vi "总磷总氮测量数据储存.vi"   [LabVIEW 2016, in "斯坦道氨氮.lvlib"]
types:
  T1 = enum16{"水样测试", "标样核查", "跨度核查", "零点核查", "加标回收", "空白测试", "平行样"}
  T2 = enum16{"维护数据", "水样测试", "标样核查", "零点核查", "跨度核查", "空白测试", "平行样测试", "加标回收", "空白校准", "标样校准", "初始化（清洗）"}
  T3 = cluster{"时间标识":timestamp, "测量模式":enum16{"维护数据", "水样测试", "标样核查", "零点核查", "跨度核查", "空白测试", "平行样测试", "加标回收", "空白校准", "标样校准", "初始化（清洗）"}, "数据标记表":string, "监测值":sgl, "单位":u16, "数据标识":string, "因子编码":u32, "标样参考值":sgl, "F0":sgl, "F1":sgl, "F2":sgl, "F3":sgl, "F4":sgl, "F5":sgl, "F6":sgl, "F7":sgl, "X":sgl, "温度":sgl, "湿度":sgl, "量程标识":string, "SN":string, "跨度值":sgl}
  T4 = cluster{"运行模式":enum16{"维护模式", "常规模式", "应急模式", "质控模式"}, "质控频次":enum16{"关闭", "每天", "星期一", "星期二", "星期三", "星期四", "星期五", "星期六", "星期日"}, "空白核查时间":u16, "跨度核查时间":u16, "24H周期设置":bool[]}
  T5 = cluster{"系统时间":timestamp, "工作状态":u16, "测量模式":enum16{"待机", "连续模式", "周期模式", "定点模式", "受控模式", "手动模式"}, "告警代码":u16, "故障代码":u16, "日志代码":u16, "软件版本":u16, "F0":sgl, "F1":sgl, "F2":sgl, "F3":sgl, "T":sgl, "H":sgl, "id":u16, "flowid":u16, "量程":u16, "总磷控温温度1":sgl, "营养盐控温温度2":sgl, "ADC":sgl}
  T6 = cluster{"因子编码":u32, "单位":u16, "标样参考值":sgl, "水样数据时间":timestamp, "水样实测值":sgl, "水样数据标识":string, "标样数据时间":timestamp, "标样实测值":sgl, "标样数据标识":string, "空白数据时间":timestamp, "空白实测值":sgl, "空白数据标识":string, "零点核查数据时间":timestamp, "零点核查实测值":sgl, "零点核查数据标识":string, "跨度核查数据时间":timestamp, "跨度核查实测值":sgl, "跨度核查数据标识":string, "加标回收数据时间":timestamp, "加标回收实测值":sgl, "加标回收数据标识":string, "平行样数据时间":timestamp, "平行样实测值":sgl, "平行样数据标识":string, "F0":sgl, "F1":sgl, "F2":sgl, "F3":sgl, "F4":sgl, "F5":sgl, "F6":sgl, "F7":sgl, "温度":sgl, "湿度":sgl, "X值":sgl, "fidrange":u16}[]
  T7 = cluster{"因子编码":u32, "单位":u16, "标样参考值":sgl, "水样数据时间":timestamp, "水样实测值":sgl, "水样数据标识":string, "标样数据时间":timestamp, "标样实测值":sgl, "标样数据标识":string, "空白数据时间":timestamp, "空白实测值":sgl, "空白数据标识":string, "零点核查数据时间":timestamp, "零点核查实测值":sgl, "零点核查数据标识":string, "跨度核查数据时间":timestamp, "跨度核查实测值":sgl, "跨度核查数据标识":string, "加标回收数据时间":timestamp, "加标回收实测值":sgl, "加标回收数据标识":string, "平行样数据时间":timestamp, "平行样实测值":sgl, "平行样数据标识":string, "F0":sgl, "F1":sgl, "F2":sgl, "F3":sgl, "F4":sgl, "F5":sgl, "F6":sgl, "F7":sgl, "温度":sgl, "湿度":sgl, "X值":sgl, "fidrange":u16}
  T8 = cluster{"总磷跨度值":dbl, "总磷零点标准液浓度":dbl, "总磷跨度标准液浓度":dbl, "总磷标准液标准浓度":dbl, "总氮跨度值":dbl, "总氮零点标准液浓度":dbl, "总氮跨度标准液浓度":dbl, "总氮标准液标准浓度":dbl, "COD跨度值":dbl, "COD零点标准液浓度":dbl, "COD跨度标准液浓度":dbl, "COD标准液标准浓度":dbl, "氨氮跨度值":dbl, "氨氮零点标准液浓度":dbl, "氨氮跨度标准液浓度":dbl, "氨氮标准液标准浓度":dbl, "磷酸盐跨度值":dbl, "磷酸盐零点标准液浓度":dbl, "磷酸盐跨度标准液浓度":dbl, "磷酸盐标准液标准浓度":dbl, "硝氮跨度值":dbl, "硝氮零点标准液浓度":dbl, "硝氮跨度标准液浓度":dbl, "硝氮标准液标准浓度":dbl, "亚硝氮跨度值":dbl, "亚硝氮零点标准液浓度":dbl, "亚硝氮跨度标准液浓度":dbl, "亚硝氮标准液标准浓度":dbl, "硫化物跨度值":dbl, "硫化物零点标准液浓度":dbl, "硫化物跨度标准液浓度":dbl, "硫化物标准液标准浓度":dbl, "硅酸盐跨度值":dbl, "硅酸盐零点标准液浓度":dbl, "硅酸盐跨度标准液浓度":dbl, "硅酸盐标准液标准浓度":dbl}
  T9 = typedef "斯坦道氨氮.lvlib/关键参数.ctl" = cluster{"测量量程":sgl, "测量检出限":sgl, "测量精度":sgl, "测量间隔":sgl, "消解温度":sgl, "消解时长":sgl, "三项式系数":sgl, "二次多项式系数":sgl, "曲线斜率":sgl, "曲线截距":sgl, "线性相关系数":sgl, "空白校准时间":timestamp, "标样校准时间":timestamp, "测量信号值":sgl, "稀释倍数":sgl, "量程系数":sgl}
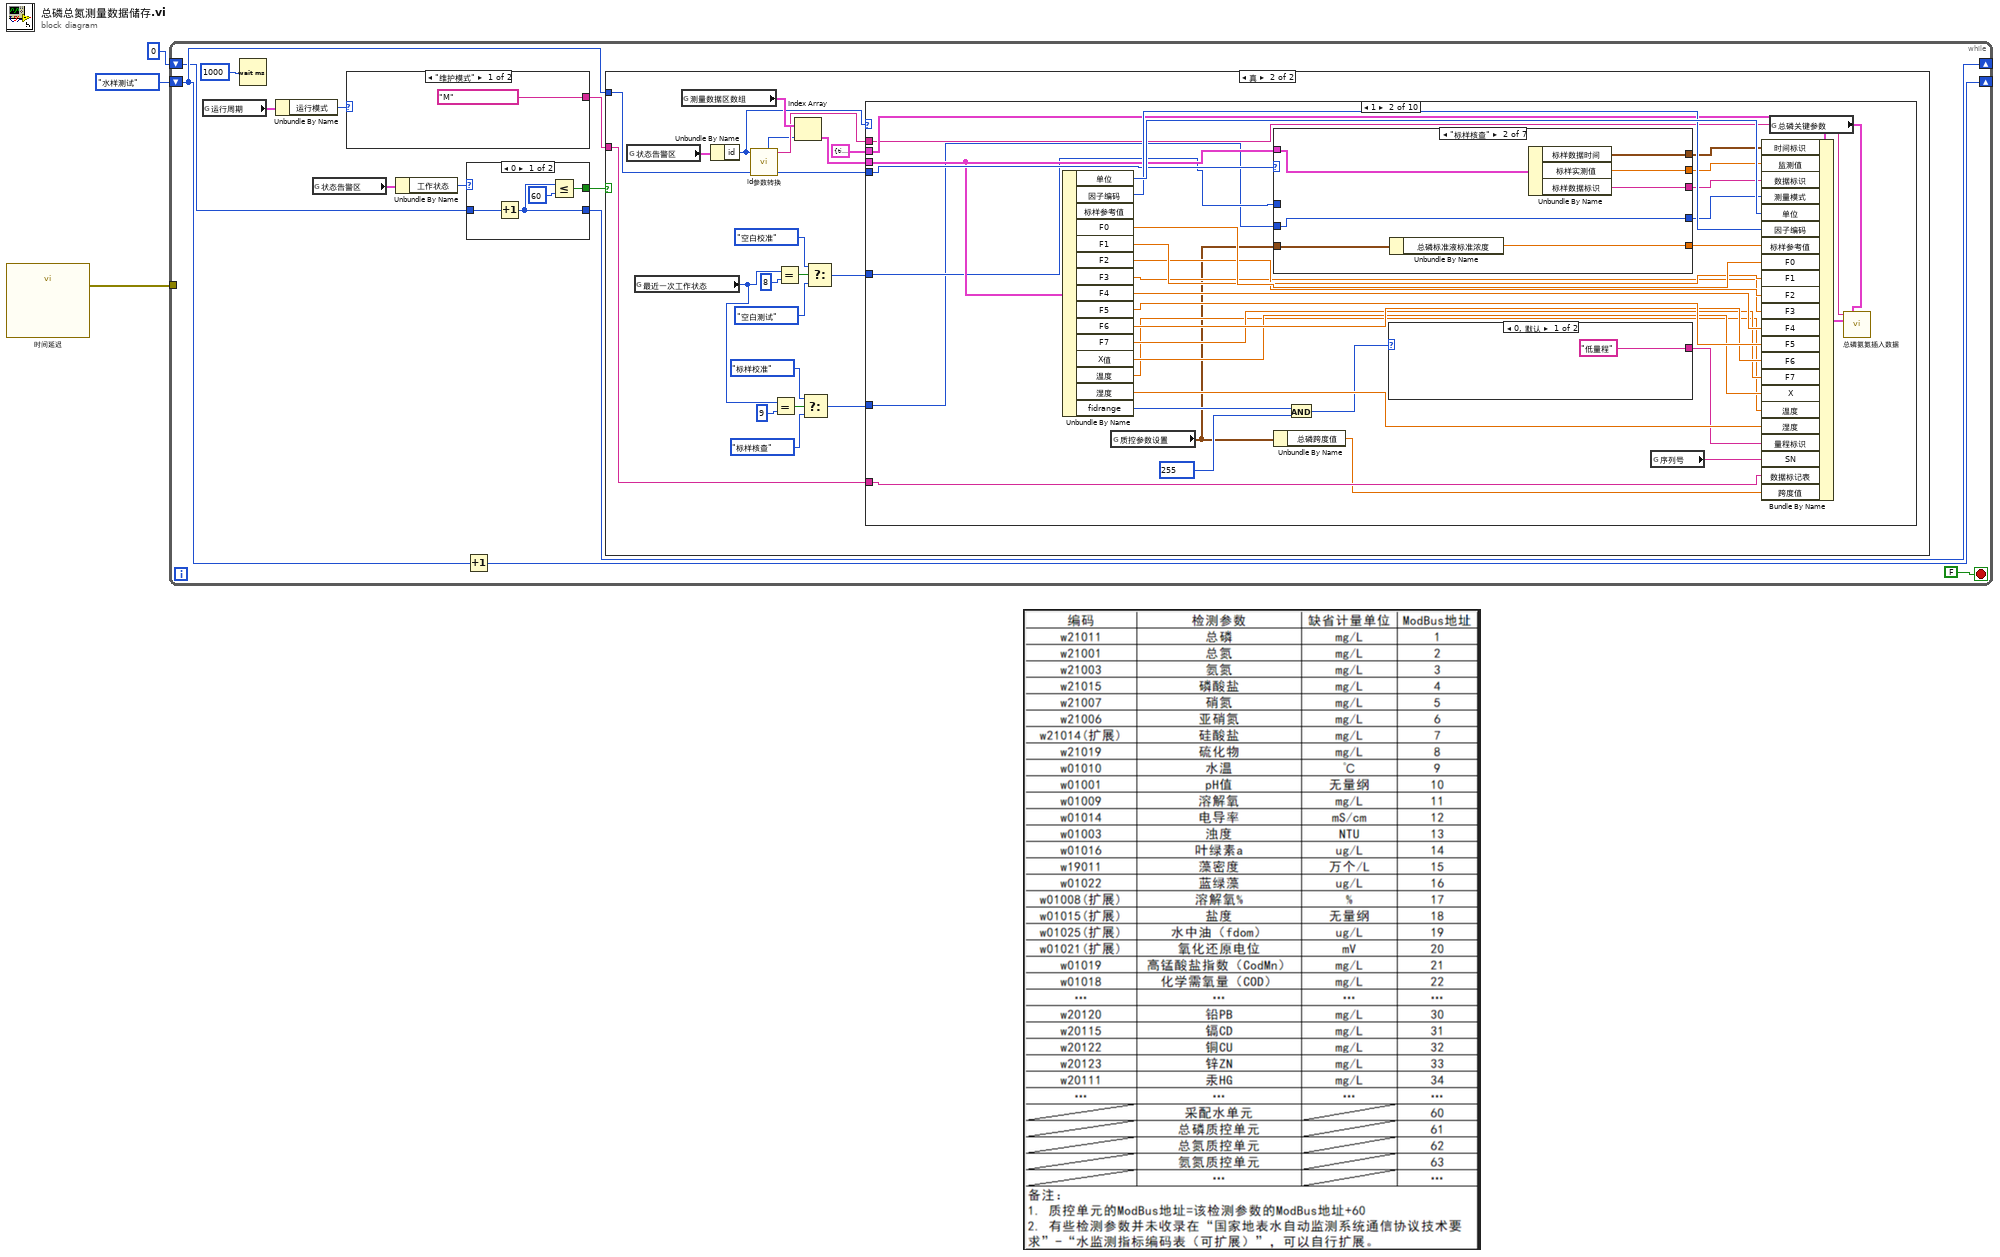
[diagram p0: block diagram]
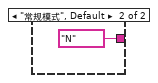
[diagram p3: hidden frame]
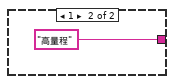
[diagram p6: hidden frame]
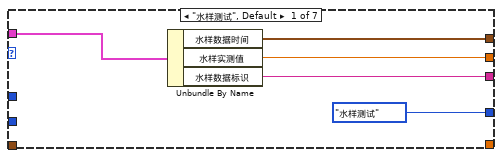
[diagram p7: hidden frame]
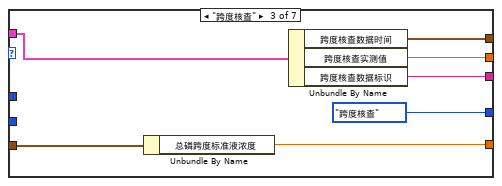
[diagram p8: hidden frame]
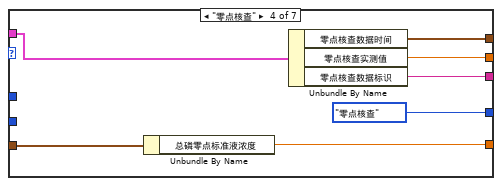
[diagram p9: hidden frame]
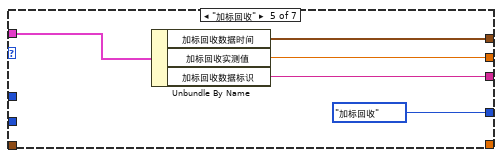
[diagram p10: hidden frame]
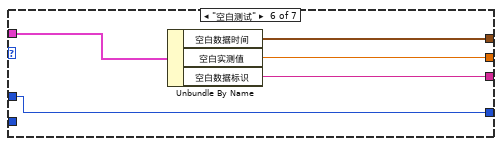
[diagram p11: hidden frame]
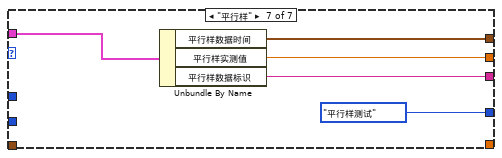
[diagram p12: hidden frame]
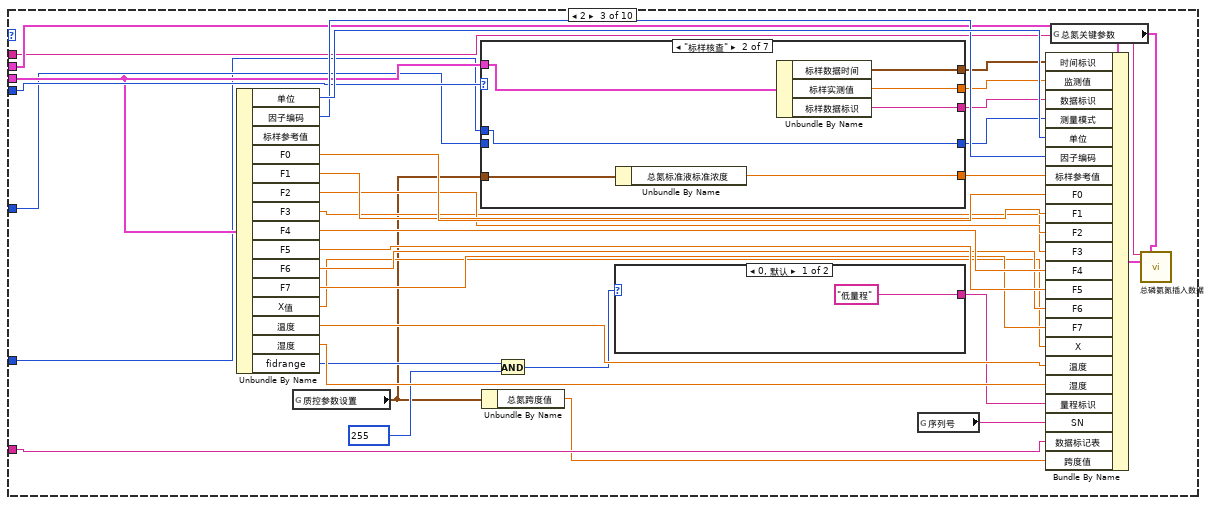
[diagram p13: hidden frame]
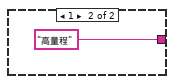
[diagram p14: hidden frame]
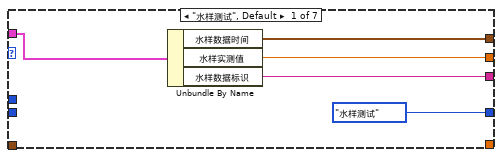
[diagram p15: hidden frame]
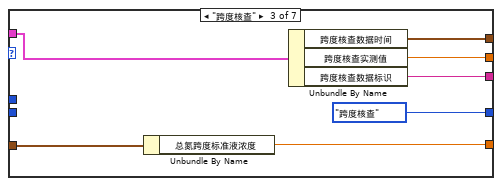
[diagram p16: hidden frame]
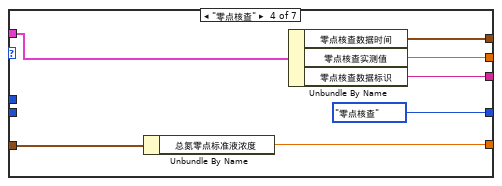
[diagram p17: hidden frame]
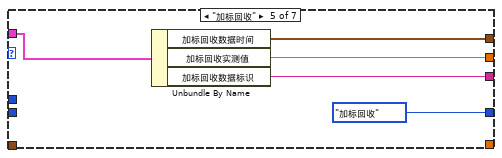
[diagram p18: hidden frame]
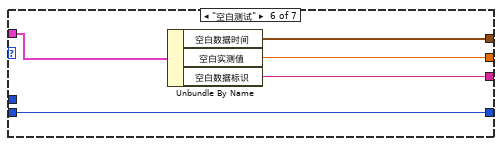
[diagram p19: hidden frame]
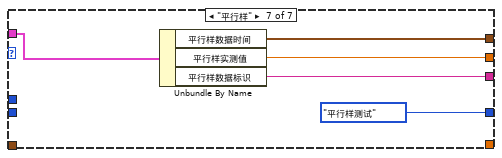
[diagram p20: hidden frame]
diagram:
  n1 = call "时间延迟"() -> ("error out"=w1:errorcluster)  [unwired: 11 in]
  n2 = while {
    shift-right: [w13] -> _
    shift-left: T1."水样测试" ("测量模式") -> [w12]
    shift-right: [w6] -> _
    shift-left: u32 0 ("等待时间（毫秒）") -> [w7]
    tunnel: w1 -> [_]
    stop <- FALSE stop-if-true
    n3 = global read "总磷总氮断电保存全局变量.vi" "运行周期"() -> (w11:T4)
    n4 = Wait (ms)(milliseconds to wait=u32 1000 ("等待时间（毫秒）")) -> ()  [unwired: 1 out]
    n5 = Unbundle By Name(w11) -> ("运行模式"=w10:enum16{"维护模式", "常规模式", "应急模式", "质控模式"})
    n6 = global read "VAR总磷总氮全局变量.vi" "状态告警区"() -> (w9:T5)
    n7 = case shown="\"维护模式\"" w10 {
      tunnel: ["M" ("数据标记表") "N" ("数据标记表")] -> w14
      frame "维护模式" {
      }
      frame "常规模式", Default {
      }
    }
    n8 = Unbundle By Name(w9) -> ("工作状态"=w8:u16)
    n9 = Increment(x=w12) -> (x+1=w13:T1)
    n10 = case shown="0" w8 {
      tunnel: w7 -> [w19 _]
      tunnel: [w18 _] -> w6
      tunnel: [w16 _] -> w5
      frame 0 {
        n11 = Increment(x=w19) -> (x+1=w18:u32)
        n12 = Less Or Equal?(x=w18, y=u32 60) -> (x <= y?=w16:bool)
      }
      frame 1, Default {
      }
    }
    n13 = case shown="真" w5 {
      tunnel: w14 -> [_ w41]
      tunnel: w12 -> [_ w40]
      frame False {
      }
      frame True {
        n14 = global read "VAR总磷总氮全局变量.vi" "状态告警区"() -> (w39:T5)
        n15 = global read "VAR总磷总氮全局变量.vi" "最近一次工作状态"() -> (w24:u16)
        n16 = global read "VAR总磷总氮全局变量.vi" "测量数据区数组"() -> (w37:T6)
        n17 = Unbundle By Name(w39) -> ("id"=w35:u16)
        n18 = call "id参数转换.vi"("id"=w35) -> ("table输出"=w34:string, "数组资源索引"=w33:i32)  [unwired: 9 in]
        n19 = Equal?(x=w24, y=u16 9) -> (x = y?=w26:bool)
        n20 = Equal?(x=w24, y=u16 8) -> (x = y?=w31:bool)
        n21 = Index Array(array=w37, index=w33) -> (element=w36:T7)
        n22 = Select(t=T2."标样校准" ("测量模式"), s=w26, f=T2."标样核查" ("测量模式")) -> (s? t:f=w22:T2)
        n23 = Select(t=T2."空白校准" ("测量模式"), s=w31, f=T2."空白测试" ("测量模式")) -> (s? t:f=w23:T2)
        n24 = case shown="1" w35 {
          tunnel: w41 -> [_ w51 w128 w206 w283 w360 w437 w514 w591 w668]
          tunnel: w40 -> [_ w59 w139 w216 w293 w370 w447 w524 w601 w678]
          tunnel: T3 {"时间标识"=timestamp(0 s since 1904-01-01), "测量模式"=enum."水样测试", "数据标记表"="N", "监测值"=0.0, "单位"=0, "数据标识"="", "因子编码"=0, "标样参考值"=0.0, "F0"=0.0, "F1"=0.0, "F2"=0.0, "F3"=0.0, "F4"=0.0, "F5"=0.0, "F6"=0.0, "F7"=0.0, "X"=0.0, "温度"=0.0, "湿度"=0.0, "量程标识"="", "SN"="", "跨度值"=0.0} ("data") -> [_ w49 w126 w204 w281 w358 w435 w512 w589 w666]
          tunnel: w36 -> [_ w46 w123 w201 w278 w355 w432 w509 w586 w662]
          tunnel: w34 -> [_ w45 w122 w199 w276 w353 w430 w507 w584 w661]
          tunnel: w23 -> [_ w44 w121 w197 w275 w352 w429 w505 w583 w660]
          tunnel: w22 -> [_ w43 w120 w198 w274 w351 w428 w506 w582 w659]
          frame Default {
          }
          frame 1 {
            n25 = Unbundle By Name(w46) -> ("单位"=w75:u16, "因子编码"=w74:u32, "F0"=w73:sgl, "F1"=w72:sgl, "F2"=w71:sgl, "F3"=w70:sgl, "F4"=w69:sgl, "F5"=w68:sgl, "F6"=w67:sgl, "F7"=w66:sgl, "X值"=w65:sgl, "温度"=w64:sgl, "湿度"=w63:sgl, "fidrange"=w57:u16)  [unwired: 1 out]
            n26 = global read "总磷总氮断电保存全局变量.vi" "质控参数设置"() -> (w48:T8)
            n27 = case shown="\"标样核查\"" w59 {
              tunnel: w46 -> [w82 w89 w96 w103 w108 w113 w118]
              tunnel: [w81 w88 w95 w102 w107 w112 w117] -> w60
              tunnel: [w80 w87 w94 w101 w106 w111 w116] -> w61
              tunnel: [w79 w86 w93 w100 w105 w110 w115] -> w62
              tunnel: [T2."水样测试" ("测量模式") w83 T2."跨度核查" ("测量模式") T2."零点核查" ("测量模式") T2."加标回收" ("测量模式") w109 T2."平行样测试" ("测量模式")] -> w50
              tunnel: w48 -> [_ w85 w91 w98 _ _ _]
              tunnel: [_ w84 w90 w97 _ _ _] -> w58
              tunnel: w44 -> [_ _ _ _ _ w109 _]
              tunnel: w43 -> [_ w83 _ _ _ _ _]
              frame "水样测试", Default {
                n28 = Unbundle By Name(w82) -> ("水样数据时间"=w81:timestamp, "水样实测值"=w80:sgl, "水样数据标识"=w79:string)
              }
              frame "标样核查" {
                n29 = Unbundle By Name(w85) -> ("总磷标准液标准浓度"=w84:dbl)
                n30 = Unbundle By Name(w89) -> ("标样数据时间"=w88:timestamp, "标样实测值"=w87:sgl, "标样数据标识"=w86:string)
              }
              frame "跨度核查" {
                n31 = Unbundle By Name(w91) -> ("总磷跨度标准液浓度"=w90:dbl)
                n32 = Unbundle By Name(w96) -> ("跨度核查数据时间"=w95:timestamp, "跨度核查实测值"=w94:sgl, "跨度核查数据标识"=w93:string)
              }
              frame "零点核查" {
                n33 = Unbundle By Name(w98) -> ("总磷零点标准液浓度"=w97:dbl)
                n34 = Unbundle By Name(w103) -> ("零点核查数据时间"=w102:timestamp, "零点核查实测值"=w101:sgl, "零点核查数据标识"=w100:string)
              }
              frame "加标回收" {
                n35 = Unbundle By Name(w108) -> ("加标回收数据时间"=w107:timestamp, "加标回收实测值"=w106:sgl, "加标回收数据标识"=w105:string)
              }
              frame "空白测试" {
                n36 = Unbundle By Name(w113) -> ("空白数据时间"=w112:timestamp, "空白实测值"=w111:sgl, "空白数据标识"=w110:string)
              }
              frame "平行样" {
                n37 = Unbundle By Name(w118) -> ("平行样数据时间"=w117:timestamp, "平行样实测值"=w116:sgl, "平行样数据标识"=w115:string)
              }
            }
            n38 = Unbundle By Name(w48) -> ("总磷跨度值"=w47:dbl)
            n39 = And(x=w57, y=u16 255) -> (x .and. y?=w55:u16)
            n40 = case shown="0, 默认" w55 {
              tunnel: ["低量程" ("格式字符串") "高量程" ("格式字符串")] -> w54
              frame 0, Default {
              }
              frame 1 {
              }
            }
            n41 = global read "VAR总磷总氮全局变量.vi" "序列号"() -> (w52:string)
            n42 = Bundle By Name(cluster=w49, "时间标识"=w60, "监测值"=w61, "数据标识"=w62, "测量模式"=w50, "单位"=w75, "因子编码"=w74, "标样参考值"=w58, "F0"=w73, "F1"=w72, "F2"=w71, "F3"=w70, "F4"=w69, "F5"=w68, "F6"=w67, "F7"=w66, "X"=w65, "温度"=w64, "湿度"=w63, "量程标识"=w54, "SN"=w52, "数据标记表"=w51, "跨度值"=w47) -> (w53:T3)
            n43 = global read "VAR总磷总氮全局变量.vi" "总磷关键参数"() -> (w42:T9)
            n44 = call "总磷氨氮插入数据.vi"("table"=w45, "关键参数"=w42, "data"=w53) -> ()  [unwired: 12 in, 1 out]
          }
          frame 2 {
            n45 = Unbundle By Name(w123) -> ("单位"=w152:u16, "因子编码"=w151:u32, "F0"=w150:sgl, "F1"=w149:sgl, "F2"=w148:sgl, "F3"=w147:sgl, "F4"=w146:sgl, "F5"=w145:sgl, "F6"=w144:sgl, "F7"=w143:sgl, "X值"=w142:sgl, "温度"=w141:sgl, "湿度"=w140:sgl, "fidrange"=w132:u16)  [unwired: 1 out]
            n46 = global read "总磷总氮断电保存全局变量.vi" "质控参数设置"() -> (w125:T8)
            n47 = case shown="\"标样核查\"" w139 {
              tunnel: w123 -> [w159 w166 w173 w180 w185 w190 w195]
              tunnel: [w158 w165 w172 w179 w184 w189 w194] -> w138
              tunnel: [w157 w164 w171 w178 w183 w188 w193] -> w137
              tunnel: [w156 w163 w170 w177 w182 w187 w192] -> w136
              tunnel: [T2."水样测试" ("测量模式") w160 T2."跨度核查" ("测量模式") T2."零点核查" ("测量模式") T2."加标回收" ("测量模式") w186 T2."平行样测试" ("测量模式")] -> w127
              tunnel: w125 -> [_ w162 w168 w175 _ _ _]
              tunnel: [_ w161 w167 w174 _ _ _] -> w135
              tunnel: w121 -> [_ _ _ _ _ w186 _]
              tunnel: w120 -> [_ w160 _ _ _ _ _]
              frame "水样测试", Default {
                n48 = Unbundle By Name(w159) -> ("水样数据时间"=w158:timestamp, "水样实测值"=w157:sgl, "水样数据标识"=w156:string)
              }
              frame "标样核查" {
                n49 = Unbundle By Name(w162) -> ("总氮标准液标准浓度"=w161:dbl)
                n50 = Unbundle By Name(w166) -> ("标样数据时间"=w165:timestamp, "标样实测值"=w164:sgl, "标样数据标识"=w163:string)
              }
              frame "跨度核查" {
                n51 = Unbundle By Name(w168) -> ("总氮跨度标准液浓度"=w167:dbl)
                n52 = Unbundle By Name(w173) -> ("跨度核查数据时间"=w172:timestamp, "跨度核查实测值"=w171:sgl, "跨度核查数据标识"=w170:string)
              }
              frame "零点核查" {
                n53 = Unbundle By Name(w175) -> ("总氮零点标准液浓度"=w174:dbl)
                n54 = Unbundle By Name(w180) -> ("零点核查数据时间"=w179:timestamp, "零点核查实测值"=w178:sgl, "零点核查数据标识"=w177:string)
              }
              frame "加标回收" {
                n55 = Unbundle By Name(w185) -> ("加标回收数据时间"=w184:timestamp, "加标回收实测值"=w183:sgl, "加标回收数据标识"=w182:string)
              }
              frame "空白测试" {
                n56 = Unbundle By Name(w190) -> ("空白数据时间"=w189:timestamp, "空白实测值"=w188:sgl, "空白数据标识"=w187:string)
              }
              frame "平行样" {
                n57 = Unbundle By Name(w195) -> ("平行样数据时间"=w194:timestamp, "平行样实测值"=w193:sgl, "平行样数据标识"=w192:string)
              }
            }
            n58 = Unbundle By Name(w125) -> ("总氮跨度值"=w124:dbl)
            n59 = And(x=w132, y=u16 255) -> (x .and. y?=w133:u16)
            n60 = case shown="0, 默认" w133 {
              tunnel: ["低量程" ("格式字符串") "高量程" ("格式字符串")] -> w131
              frame 0, Default {
              }
              frame 1 {
              }
            }
            n61 = global read "VAR总磷总氮全局变量.vi" "序列号"() -> (w129:string)
            n62 = Bundle By Name(cluster=w126, "时间标识"=w138, "监测值"=w137, "数据标识"=w136, "测量模式"=w127, "单位"=w152, "因子编码"=w151, "标样参考值"=w135, "F0"=w150, "F1"=w149, "F2"=w148, "F3"=w147, "F4"=w146, "F5"=w145, "F6"=w144, "F7"=w143, "X"=w142, "温度"=w141, "湿度"=w140, "量程标识"=w131, "SN"=w129, "数据标记表"=w128, "跨度值"=w124) -> (w130:T3)
            n63 = global read "VAR总磷总氮全局变量.vi" "总氮关键参数"() -> (w119:T9)
            n64 = call "总磷氨氮插入数据.vi"("table"=w122, "关键参数"=w119, "data"=w130) -> ()  [unwired: 12 in, 1 out]
          }
          frame 3 {
            n65 = Unbundle By Name(w201) -> ("单位"=w229:u16, "因子编码"=w228:u32, "F0"=w227:sgl, "F1"=w226:sgl, "F2"=w225:sgl, "F3"=w224:sgl, "F4"=w223:sgl, "F5"=w222:sgl, "F6"=w221:sgl, "F7"=w220:sgl, "X值"=w219:sgl, "温度"=w218:sgl, "湿度"=w217:sgl, "fidrange"=w209:u16)  [unwired: 1 out]
            n66 = global read "总磷总氮断电保存全局变量.vi" "质控参数设置"() -> (w203:T8)
            n67 = case shown="\"空白测试\"" w216 {
              tunnel: w201 -> [w236 w243 w250 w257 w262 w267 w272]
              tunnel: [w235 w242 w249 w256 w261 w266 w271] -> w215
              tunnel: [w234 w241 w248 w255 w260 w265 w270] -> w214
              tunnel: [w233 w240 w247 w254 w259 w264 w269] -> w213
              tunnel: [T2."水样测试" ("测量模式") w237 T2."跨度核查" ("测量模式") T2."零点核查" ("测量模式") T2."加标回收" ("测量模式") w263 T2."平行样测试" ("测量模式")] -> w205
              tunnel: w203 -> [_ w239 w245 w252 _ _ _]
              tunnel: [_ w238 w244 w251 _ _ _] -> w212
              tunnel: w198 -> [_ w237 _ _ _ _ _]
              tunnel: w197 -> [_ _ _ _ _ w263 _]
              frame "水样测试", Default {
                n68 = Unbundle By Name(w236) -> ("水样数据时间"=w235:timestamp, "水样实测值"=w234:sgl, "水样数据标识"=w233:string)
              }
              frame "标样核查" {
                n69 = Unbundle By Name(w239) -> ("氨氮标准液标准浓度"=w238:dbl)
                n70 = Unbundle By Name(w243) -> ("标样数据时间"=w242:timestamp, "标样实测值"=w241:sgl, "标样数据标识"=w240:string)
              }
              frame "跨度核查" {
                n71 = Unbundle By Name(w245) -> ("氨氮跨度标准液浓度"=w244:dbl)
                n72 = Unbundle By Name(w250) -> ("跨度核查数据时间"=w249:timestamp, "跨度核查实测值"=w248:sgl, "跨度核查数据标识"=w247:string)
              }
              frame "零点核查" {
                n73 = Unbundle By Name(w252) -> ("氨氮零点标准液浓度"=w251:dbl)
                n74 = Unbundle By Name(w257) -> ("零点核查数据时间"=w256:timestamp, "零点核查实测值"=w255:sgl, "零点核查数据标识"=w254:string)
              }
              frame "加标回收" {
                n75 = Unbundle By Name(w262) -> ("加标回收数据时间"=w261:timestamp, "加标回收实测值"=w260:sgl, "加标回收数据标识"=w259:string)
              }
              frame "空白测试" {
                n76 = Unbundle By Name(w267) -> ("空白数据时间"=w266:timestamp, "空白实测值"=w265:sgl, "空白数据标识"=w264:string)
              }
              frame "平行样" {
                n77 = Unbundle By Name(w272) -> ("平行样数据时间"=w271:timestamp, "平行样实测值"=w270:sgl, "平行样数据标识"=w269:string)
              }
            }
            n78 = Unbundle By Name(w203) -> ("氨氮跨度值"=w202:dbl)
            n79 = And(x=w209, y=u16 255) -> (x .and. y?=w210:u16)
            n80 = case shown="0, 默认" w210 {
              tunnel: ["低量程" ("格式字符串") "高量程" ("格式字符串")] -> w208
              frame 0, Default {
              }
              frame 1 {
              }
            }
            n81 = global read "VAR总磷总氮全局变量.vi" "序列号"() -> (w207:string)
            n82 = Bundle By Name(cluster=w204, "时间标识"=w215, "监测值"=w214, "数据标识"=w213, "测量模式"=w205, "单位"=w229, "因子编码"=w228, "标样参考值"=w212, "F0"=w227, "F1"=w226, "F2"=w225, "F3"=w224, "F4"=w223, "F5"=w222, "F6"=w221, "F7"=w220, "X"=w219, "温度"=w218, "湿度"=w217, "量程标识"=w208, "SN"=w207, "数据标记表"=w206, "跨度值"=w202) -> (w200:T3)
            n83 = global read "VAR总磷总氮全局变量.vi" "氨氮关键参数"() -> (w196:T9)
            n84 = call "总磷氨氮插入数据.vi"("table"=w199, "关键参数"=w196, "data"=w200) -> ()  [unwired: 12 in, 1 out]
          }
          frame 4 {
            n85 = Unbundle By Name(w278) -> ("单位"=w306:u16, "因子编码"=w305:u32, "F0"=w304:sgl, "F1"=w303:sgl, "F2"=w302:sgl, "F3"=w301:sgl, "F4"=w300:sgl, "F5"=w299:sgl, "F6"=w298:sgl, "F7"=w297:sgl, "X值"=w296:sgl, "温度"=w295:sgl, "湿度"=w294:sgl, "fidrange"=w286:u16)  [unwired: 1 out]
            n86 = global read "总磷总氮断电保存全局变量.vi" "质控参数设置"() -> (w280:T8)
            n87 = Unbundle By Name(w280) -> ("磷酸盐跨度值"=w279:dbl)
            n88 = case shown="\"标样核查\"" w293 {
              tunnel: w278 -> [w313 w320 w327 w334 w339 w344 w349]
              tunnel: [w312 w319 w326 w333 w338 w343 w348] -> w292
              tunnel: [w311 w318 w325 w332 w337 w342 w347] -> w291
              tunnel: [w310 w317 w324 w331 w336 w341 w346] -> w290
              tunnel: [T2."水样测试" ("测量模式") w314 T2."跨度核查" ("测量模式") T2."零点核查" ("测量模式") T2."加标回收" ("测量模式") w340 T2."平行样测试" ("测量模式")] -> w282
              tunnel: w280 -> [_ w316 w322 w329 _ _ _]
              tunnel: [_ w315 w321 w328 _ _ _] -> w289
              tunnel: w275 -> [_ _ _ _ _ w340 _]
              tunnel: w274 -> [_ w314 _ _ _ _ _]
              frame "水样测试", Default {
                n89 = Unbundle By Name(w313) -> ("水样数据时间"=w312:timestamp, "水样实测值"=w311:sgl, "水样数据标识"=w310:string)
              }
              frame "标样核查" {
                n90 = Unbundle By Name(w316) -> ("磷酸盐标准液标准浓度"=w315:dbl)
                n91 = Unbundle By Name(w320) -> ("标样数据时间"=w319:timestamp, "标样实测值"=w318:sgl, "标样数据标识"=w317:string)
              }
              frame "跨度核查" {
                n92 = Unbundle By Name(w322) -> ("磷酸盐跨度标准液浓度"=w321:dbl)
                n93 = Unbundle By Name(w327) -> ("跨度核查数据时间"=w326:timestamp, "跨度核查实测值"=w325:sgl, "跨度核查数据标识"=w324:string)
              }
              frame "零点核查" {
                n94 = Unbundle By Name(w329) -> ("磷酸盐零点标准液浓度"=w328:dbl)
                n95 = Unbundle By Name(w334) -> ("零点核查数据时间"=w333:timestamp, "零点核查实测值"=w332:sgl, "零点核查数据标识"=w331:string)
              }
              frame "加标回收" {
                n96 = Unbundle By Name(w339) -> ("加标回收数据时间"=w338:timestamp, "加标回收实测值"=w337:sgl, "加标回收数据标识"=w336:string)
              }
              frame "空白测试" {
                n97 = Unbundle By Name(w344) -> ("空白数据时间"=w343:timestamp, "空白实测值"=w342:sgl, "空白数据标识"=w341:string)
              }
              frame "平行样" {
                n98 = Unbundle By Name(w349) -> ("平行样数据时间"=w348:timestamp, "平行样实测值"=w347:sgl, "平行样数据标识"=w346:string)
              }
            }
            n99 = And(x=w286, y=u16 255) -> (x .and. y?=w287:u16)
            n100 = case shown="0, 默认" w287 {
              tunnel: ["低量程" ("格式字符串") "高量程" ("格式字符串")] -> w285
              frame 0, Default {
              }
              frame 1 {
              }
            }
            n101 = global read "VAR总磷总氮全局变量.vi" "序列号"() -> (w284:string)
            n102 = Bundle By Name(cluster=w281, "时间标识"=w292, "监测值"=w291, "数据标识"=w290, "测量模式"=w282, "单位"=w306, "因子编码"=w305, "标样参考值"=w289, "F0"=w304, "F1"=w303, "F2"=w302, "F3"=w301, "F4"=w300, "F5"=w299, "F6"=w298, "F7"=w297, "X"=w296, "温度"=w295, "湿度"=w294, "量程标识"=w285, "SN"=w284, "数据标记表"=w283, "跨度值"=w279) -> (w277:T3)
            n103 = global read "VAR总磷总氮全局变量.vi" "磷酸盐关键参数"() -> (w273:T9)
            n104 = call "总磷氨氮插入数据.vi"("table"=w276, "关键参数"=w273, "data"=w277) -> ()  [unwired: 12 in, 1 out]
          }
          frame 5 {
            n105 = Unbundle By Name(w355) -> ("单位"=w383:u16, "因子编码"=w382:u32, "F0"=w381:sgl, "F1"=w380:sgl, "F2"=w379:sgl, "F3"=w378:sgl, "F4"=w377:sgl, "F5"=w376:sgl, "F6"=w375:sgl, "F7"=w374:sgl, "X值"=w373:sgl, "温度"=w372:sgl, "湿度"=w371:sgl, "fidrange"=w363:u16)  [unwired: 1 out]
            n106 = global read "总磷总氮断电保存全局变量.vi" "质控参数设置"() -> (w357:T8)
            n107 = case shown="\"标样核查\"" w370 {
              tunnel: w355 -> [w390 w397 w404 w411 w416 w421 w426]
              tunnel: [w389 w396 w403 w410 w415 w420 w425] -> w369
              tunnel: [w388 w395 w402 w409 w414 w419 w424] -> w368
              tunnel: [w387 w394 w401 w408 w413 w418 w423] -> w367
              tunnel: [T2."水样测试" ("测量模式") w391 T2."跨度核查" ("测量模式") T2."零点核查" ("测量模式") T2."加标回收" ("测量模式") w417 T2."平行样测试" ("测量模式")] -> w359
              tunnel: w357 -> [_ w393 w399 w406 _ _ _]
              tunnel: [_ w392 w398 w405 _ _ _] -> w366
              tunnel: w352 -> [_ _ _ _ _ w417 _]
              tunnel: w351 -> [_ w391 _ _ _ _ _]
              frame "水样测试", Default {
                n108 = Unbundle By Name(w390) -> ("水样数据时间"=w389:timestamp, "水样实测值"=w388:sgl, "水样数据标识"=w387:string)
              }
              frame "标样核查" {
                n109 = Unbundle By Name(w393) -> ("硝氮标准液标准浓度"=w392:dbl)
                n110 = Unbundle By Name(w397) -> ("标样数据时间"=w396:timestamp, "标样实测值"=w395:sgl, "标样数据标识"=w394:string)
              }
              frame "跨度核查" {
                n111 = Unbundle By Name(w399) -> ("硝氮跨度标准液浓度"=w398:dbl)
                n112 = Unbundle By Name(w404) -> ("跨度核查数据时间"=w403:timestamp, "跨度核查实测值"=w402:sgl, "跨度核查数据标识"=w401:string)
              }
              frame "零点核查" {
                n113 = Unbundle By Name(w406) -> ("硝氮零点标准液浓度"=w405:dbl)
                n114 = Unbundle By Name(w411) -> ("零点核查数据时间"=w410:timestamp, "零点核查实测值"=w409:sgl, "零点核查数据标识"=w408:string)
              }
              frame "加标回收" {
                n115 = Unbundle By Name(w416) -> ("加标回收数据时间"=w415:timestamp, "加标回收实测值"=w414:sgl, "加标回收数据标识"=w413:string)
              }
              frame "空白测试" {
                n116 = Unbundle By Name(w421) -> ("空白数据时间"=w420:timestamp, "空白实测值"=w419:sgl, "空白数据标识"=w418:string)
              }
              frame "平行样" {
                n117 = Unbundle By Name(w426) -> ("平行样数据时间"=w425:timestamp, "平行样实测值"=w424:sgl, "平行样数据标识"=w423:string)
              }
            }
            n118 = Unbundle By Name(w357) -> ("硝氮跨度值"=w356:dbl)
            n119 = And(x=w363, y=u16 255) -> (x .and. y?=w364:u16)
            n120 = case shown="0, 默认" w364 {
              tunnel: ["低量程" ("格式字符串") "高量程" ("格式字符串")] -> w362
              frame 0, Default {
              }
              frame 1 {
              }
            }
            n121 = global read "VAR总磷总氮全局变量.vi" "序列号"() -> (w361:string)
            n122 = Bundle By Name(cluster=w358, "时间标识"=w369, "监测值"=w368, "数据标识"=w367, "测量模式"=w359, "单位"=w383, "因子编码"=w382, "标样参考值"=w366, "F0"=w381, "F1"=w380, "F2"=w379, "F3"=w378, "F4"=w377, "F5"=w376, "F6"=w375, "F7"=w374, "X"=w373, "温度"=w372, "湿度"=w371, "量程标识"=w362, "SN"=w361, "数据标记表"=w360, "跨度值"=w356) -> (w354:T3)
            n123 = global read "VAR总磷总氮全局变量.vi" "硝氮关键参数"() -> (w350:T9)
            n124 = call "总磷氨氮插入数据.vi"("table"=w353, "关键参数"=w350, "data"=w354) -> ()  [unwired: 12 in, 1 out]
          }
          frame 6 {
            n125 = Unbundle By Name(w432) -> ("单位"=w460:u16, "因子编码"=w459:u32, "F0"=w458:sgl, "F1"=w457:sgl, "F2"=w456:sgl, "F3"=w455:sgl, "F4"=w454:sgl, "F5"=w453:sgl, "F6"=w452:sgl, "F7"=w451:sgl, "X值"=w450:sgl, "温度"=w449:sgl, "湿度"=w448:sgl, "fidrange"=w440:u16)  [unwired: 1 out]
            n126 = global read "总磷总氮断电保存全局变量.vi" "质控参数设置"() -> (w434:T8)
            n127 = Unbundle By Name(w434) -> ("亚硝氮跨度值"=w433:dbl)
            n128 = case shown="\"标样核查\"" w447 {
              tunnel: w432 -> [w467 w474 w481 w488 w493 w498 w503]
              tunnel: [w466 w473 w480 w487 w492 w497 w502] -> w446
              tunnel: [w465 w472 w479 w486 w491 w496 w501] -> w445
              tunnel: [w464 w471 w478 w485 w490 w495 w500] -> w444
              tunnel: [T2."水样测试" ("测量模式") w468 T2."跨度核查" ("测量模式") T2."零点核查" ("测量模式") T2."加标回收" ("测量模式") w494 T2."平行样测试" ("测量模式")] -> w436
              tunnel: w434 -> [_ w470 w476 w483 _ _ _]
              tunnel: [_ w469 w475 w482 _ _ _] -> w443
              tunnel: w429 -> [_ _ _ _ _ w494 _]
              tunnel: w428 -> [_ w468 _ _ _ _ _]
              frame "水样测试", Default {
                n129 = Unbundle By Name(w467) -> ("水样数据时间"=w466:timestamp, "水样实测值"=w465:sgl, "水样数据标识"=w464:string)
              }
              frame "标样核查" {
                n130 = Unbundle By Name(w470) -> ("亚硝氮标准液标准浓度"=w469:dbl)
                n131 = Unbundle By Name(w474) -> ("标样数据时间"=w473:timestamp, "标样实测值"=w472:sgl, "标样数据标识"=w471:string)
              }
              frame "跨度核查" {
                n132 = Unbundle By Name(w476) -> ("亚硝氮跨度标准液浓度"=w475:dbl)
                n133 = Unbundle By Name(w481) -> ("跨度核查数据时间"=w480:timestamp, "跨度核查实测值"=w479:sgl, "跨度核查数据标识"=w478:string)
              }
              frame "零点核查" {
                n134 = Unbundle By Name(w483) -> ("亚硝氮零点标准液浓度"=w482:dbl)
                n135 = Unbundle By Name(w488) -> ("零点核查数据时间"=w487:timestamp, "零点核查实测值"=w486:sgl, "零点核查数据标识"=w485:string)
              }
              frame "加标回收" {
                n136 = Unbundle By Name(w493) -> ("加标回收数据时间"=w492:timestamp, "加标回收实测值"=w491:sgl, "加标回收数据标识"=w490:string)
              }
              frame "空白测试" {
                n137 = Unbundle By Name(w498) -> ("空白数据时间"=w497:timestamp, "空白实测值"=w496:sgl, "空白数据标识"=w495:string)
              }
              frame "平行样" {
                n138 = Unbundle By Name(w503) -> ("平行样数据时间"=w502:timestamp, "平行样实测值"=w501:sgl, "平行样数据标识"=w500:string)
              }
            }
            n139 = And(x=w440, y=u16 255) -> (x .and. y?=w441:u16)
            n140 = case shown="0, 默认" w441 {
              tunnel: ["低量程" ("格式字符串") "高量程" ("格式字符串")] -> w439
              frame 0, Default {
              }
              frame 1 {
              }
            }
            n141 = global read "VAR总磷总氮全局变量.vi" "序列号"() -> (w438:string)
            n142 = Bundle By Name(cluster=w435, "时间标识"=w446, "监测值"=w445, "数据标识"=w444, "测量模式"=w436, "单位"=w460, "因子编码"=w459, "标样参考值"=w443, "F0"=w458, "F1"=w457, "F2"=w456, "F3"=w455, "F4"=w454, "F5"=w453, "F6"=w452, "F7"=w451, "X"=w450, "温度"=w449, "湿度"=w448, "量程标识"=w439, "SN"=w438, "数据标记表"=w437, "跨度值"=w433) -> (w431:T3)
            n143 = global read "VAR总磷总氮全局变量.vi" "亚硝氮关键参数"() -> (w427:T9)
            n144 = call "总磷氨氮插入数据.vi"("table"=w430, "关键参数"=w427, "data"=w431) -> ()  [unwired: 12 in, 1 out]
          }
          frame 7 {
            n145 = Unbundle By Name(w509) -> ("单位"=w537:u16, "因子编码"=w536:u32, "F0"=w535:sgl, "F1"=w534:sgl, "F2"=w533:sgl, "F3"=w532:sgl, "F4"=w531:sgl, "F5"=w530:sgl, "F6"=w529:sgl, "F7"=w528:sgl, "X值"=w527:sgl, "温度"=w526:sgl, "湿度"=w525:sgl, "fidrange"=w517:u16)  [unwired: 1 out]
            n146 = global read "总磷总氮断电保存全局变量.vi" "质控参数设置"() -> (w511:T8)
            n147 = Unbundle By Name(w511) -> ("硅酸盐跨度值"=w510:dbl)
            n148 = case shown="\"空白测试\"" w524 {
              tunnel: w509 -> [w544 w551 w558 w565 w570 w575 w580]
              tunnel: [w543 w550 w557 w564 w569 w574 w579] -> w523
              tunnel: [w542 w549 w556 w563 w568 w573 w578] -> w522
              tunnel: [w541 w548 w555 w562 w567 w572 w577] -> w521
              tunnel: [T2."水样测试" ("测量模式") w545 T2."跨度核查" ("测量模式") T2."零点核查" ("测量模式") T2."加标回收" ("测量模式") w571 T2."平行样测试" ("测量模式")] -> w513
              tunnel: w511 -> [_ w547 w553 w560 _ _ _]
              tunnel: [_ w546 w552 w559 _ _ _] -> w520
              tunnel: w506 -> [_ w545 _ _ _ _ _]
              tunnel: w505 -> [_ _ _ _ _ w571 _]
              frame "水样测试", Default {
                n149 = Unbundle By Name(w544) -> ("水样数据时间"=w543:timestamp, "水样实测值"=w542:sgl, "水样数据标识"=w541:string)
              }
              frame "标样核查" {
                n150 = Unbundle By Name(w547) -> ("硅酸盐标准液标准浓度"=w546:dbl)
                n151 = Unbundle By Name(w551) -> ("标样数据时间"=w550:timestamp, "标样实测值"=w549:sgl, "标样数据标识"=w548:string)
              }
              frame "跨度核查" {
                n152 = Unbundle By Name(w553) -> ("硅酸盐跨度标准液浓度"=w552:dbl)
                n153 = Unbundle By Name(w558) -> ("跨度核查数据时间"=w557:timestamp, "跨度核查实测值"=w556:sgl, "跨度核查数据标识"=w555:string)
              }
              frame "零点核查" {
                n154 = Unbundle By Name(w560) -> ("硅酸盐零点标准液浓度"=w559:dbl)
                n155 = Unbundle By Name(w565) -> ("零点核查数据时间"=w564:timestamp, "零点核查实测值"=w563:sgl, "零点核查数据标识"=w562:string)
              }
              frame "加标回收" {
                n156 = Unbundle By Name(w570) -> ("加标回收数据时间"=w569:timestamp, "加标回收实测值"=w568:sgl, "加标回收数据标识"=w567:string)
              }
              frame "空白测试" {
                n157 = Unbundle By Name(w575) -> ("空白数据时间"=w574:timestamp, "空白实测值"=w573:sgl, "空白数据标识"=w572:string)
              }
              frame "平行样" {
                n158 = Unbundle By Name(w580) -> ("平行样数据时间"=w579:timestamp, "平行样实测值"=w578:sgl, "平行样数据标识"=w577:string)
              }
            }
            n159 = And(x=w517, y=u16 255) -> (x .and. y?=w518:u16)
            n160 = case shown="0, 默认" w518 {
              tunnel: ["低量程" ("格式字符串") "高量程" ("格式字符串")] -> w516
              frame 0, Default {
              }
              frame 1 {
              }
            }
            n161 = global read "VAR总磷总氮全局变量.vi" "序列号"() -> (w515:string)
            n162 = Bundle By Name(cluster=w512, "时间标识"=w523, "监测值"=w522, "数据标识"=w521, "测量模式"=w513, "单位"=w537, "因子编码"=w536, "标样参考值"=w520, "F0"=w535, "F1"=w534, "F2"=w533, "F3"=w532, "F4"=w531, "F5"=w530, "F6"=w529, "F7"=w528, "X"=w527, "温度"=w526, "湿度"=w525, "量程标识"=w516, "SN"=w515, "数据标记表"=w514, "跨度值"=w510) -> (w508:T3)
            n163 = global read "VAR总磷总氮全局变量.vi" "硅酸盐关键参数"() -> (w504:T9)
            n164 = call "总磷氨氮插入数据.vi"("table"=w507, "关键参数"=w504, "data"=w508) -> ()  [unwired: 12 in, 1 out]
          }
          frame 8 {
            n165 = Unbundle By Name(w586) -> ("单位"=w614:u16, "因子编码"=w613:u32, "F0"=w612:sgl, "F1"=w611:sgl, "F2"=w610:sgl, "F3"=w609:sgl, "F4"=w608:sgl, "F5"=w607:sgl, "F6"=w606:sgl, "F7"=w605:sgl, "X值"=w604:sgl, "温度"=w603:sgl, "湿度"=w602:sgl, "fidrange"=w594:u16)  [unwired: 1 out]
            n166 = global read "总磷总氮断电保存全局变量.vi" "质控参数设置"() -> (w588:T8)
            n167 = Unbundle By Name(w588) -> ("硫化物跨度值"=w587:dbl)
            n168 = case shown="\"标样核查\"" w601 {
              tunnel: w586 -> [w621 w628 w635 w642 w647 w652 w657]
              tunnel: [w620 w627 w634 w641 w646 w651 w656] -> w600
              tunnel: [w619 w626 w633 w640 w645 w650 w655] -> w599
              tunnel: [w618 w625 w632 w639 w644 w649 w654] -> w598
              tunnel: [T2."水样测试" ("测量模式") w622 T2."跨度核查" ("测量模式") T2."零点核查" ("测量模式") T2."加标回收" ("测量模式") w648 T2."平行样测试" ("测量模式")] -> w590
              tunnel: w588 -> [_ w624 w630 w637 _ _ _]
              tunnel: [_ w623 w629 w636 _ _ _] -> w597
              tunnel: w583 -> [_ _ _ _ _ w648 _]
              tunnel: w582 -> [_ w622 _ _ _ _ _]
              frame "水样测试", Default {
                n169 = Unbundle By Name(w621) -> ("水样数据时间"=w620:timestamp, "水样实测值"=w619:sgl, "水样数据标识"=w618:string)
              }
              frame "标样核查" {
                n170 = Unbundle By Name(w624) -> ("硫化物标准液标准浓度"=w623:dbl)
                n171 = Unbundle By Name(w628) -> ("标样数据时间"=w627:timestamp, "标样实测值"=w626:sgl, "标样数据标识"=w625:string)
              }
              frame "跨度核查" {
                n172 = Unbundle By Name(w630) -> ("硫化物跨度标准液浓度"=w629:dbl)
                n173 = Unbundle By Name(w635) -> ("跨度核查数据时间"=w634:timestamp, "跨度核查实测值"=w633:sgl, "跨度核查数据标识"=w632:string)
              }
              frame "零点核查" {
                n174 = Unbundle By Name(w637) -> ("硫化物零点标准液浓度"=w636:dbl)
                n175 = Unbundle By Name(w642) -> ("零点核查数据时间"=w641:timestamp, "零点核查实测值"=w640:sgl, "零点核查数据标识"=w639:string)
              }
              frame "加标回收" {
                n176 = Unbundle By Name(w647) -> ("加标回收数据时间"=w646:timestamp, "加标回收实测值"=w645:sgl, "加标回收数据标识"=w644:string)
              }
              frame "空白测试" {
                n177 = Unbundle By Name(w652) -> ("空白数据时间"=w651:timestamp, "空白实测值"=w650:sgl, "空白数据标识"=w649:string)
              }
              frame "平行样" {
                n178 = Unbundle By Name(w657) -> ("平行样数据时间"=w656:timestamp, "平行样实测值"=w655:sgl, "平行样数据标识"=w654:string)
              }
            }
            n179 = And(x=w594, y=u16 255) -> (x .and. y?=w595:u16)
            n180 = case shown="0, 默认" w595 {
              tunnel: ["低量程" ("格式字符串") "高量程" ("格式字符串")] -> w593
              frame 0, Default {
              }
              frame 1 {
              }
            }
            n181 = global read "VAR总磷总氮全局变量.vi" "序列号"() -> (w592:string)
            n182 = Bundle By Name(cluster=w589, "时间标识"=w600, "监测值"=w599, "数据标识"=w598, "测量模式"=w590, "单位"=w614, "因子编码"=w613, "标样参考值"=w597, "F0"=w612, "F1"=w611, "F2"=w610, "F3"=w609, "F4"=w608, "F5"=w607, "F6"=w606, "F7"=w605, "X"=w604, "温度"=w603, "湿度"=w602, "量程标识"=w593, "SN"=w592, "数据标记表"=w591, "跨度值"=w587) -> (w585:T3)
            n183 = global read "VAR总磷总氮全局变量.vi" "硫化物关键参数"() -> (w581:T9)
            n184 = call "总磷氨氮插入数据.vi"("table"=w584, "关键参数"=w581, "data"=w585) -> ()  [unwired: 12 in, 1 out]
          }
          frame 22 {
            n185 = Unbundle By Name(w662) -> ("单位"=w691:u16, "因子编码"=w690:u32, "F0"=w689:sgl, "F1"=w688:sgl, "F2"=w687:sgl, "F3"=w686:sgl, "F4"=w685:sgl, "F5"=w684:sgl, "F6"=w683:sgl, "F7"=w682:sgl, "X值"=w681:sgl, "温度"=w680:sgl, "湿度"=w679:sgl, "fidrange"=w671:u16)  [unwired: 1 out]
            n186 = global read "总磷总氮断电保存全局变量.vi" "质控参数设置"() -> (w664:T8)
            n187 = case shown="\"标样核查\"" w678 {
              tunnel: w662 -> [w698 w705 w712 w719 w724 w729 w734]
              tunnel: [w697 w704 w711 w718 w723 w728 w733] -> w677
              tunnel: [w696 w703 w710 w717 w722 w727 w732] -> w676
              tunnel: [w695 w702 w709 w716 w721 w726 w731] -> w675
              tunnel: [T2."水样测试" ("测量模式") w699 T2."跨度核查" ("测量模式") T2."零点核查" ("测量模式") T2."加标回收" ("测量模式") w725 T2."平行样测试" ("测量模式")] -> w667
              tunnel: w664 -> [_ w701 w707 w714 _ _ _]
              tunnel: [_ w700 w706 w713 _ _ _] -> w674
              tunnel: w660 -> [_ _ _ _ _ w725 _]
              tunnel: w659 -> [_ w699 _ _ _ _ _]
              frame "水样测试", Default {
                n188 = Unbundle By Name(w698) -> ("水样数据时间"=w697:timestamp, "水样实测值"=w696:sgl, "水样数据标识"=w695:string)
              }
              frame "标样核查" {
                n189 = Unbundle By Name(w701) -> ("COD标准液标准浓度"=w700:dbl)
                n190 = Unbundle By Name(w705) -> ("标样数据时间"=w704:timestamp, "标样实测值"=w703:sgl, "标样数据标识"=w702:string)
              }
              frame "跨度核查" {
                n191 = Unbundle By Name(w707) -> ("COD跨度标准液浓度"=w706:dbl)
                n192 = Unbundle By Name(w712) -> ("跨度核查数据时间"=w711:timestamp, "跨度核查实测值"=w710:sgl, "跨度核查数据标识"=w709:string)
              }
              frame "零点核查" {
                n193 = Unbundle By Name(w714) -> ("COD零点标准液浓度"=w713:dbl)
                n194 = Unbundle By Name(w719) -> ("零点核查数据时间"=w718:timestamp, "零点核查实测值"=w717:sgl, "零点核查数据标识"=w716:string)
              }
              frame "加标回收" {
                n195 = Unbundle By Name(w724) -> ("加标回收数据时间"=w723:timestamp, "加标回收实测值"=w722:sgl, "加标回收数据标识"=w721:string)
              }
              frame "空白测试" {
                n196 = Unbundle By Name(w729) -> ("空白数据时间"=w728:timestamp, "空白实测值"=w727:sgl, "空白数据标识"=w726:string)
              }
              frame "平行样" {
                n197 = Unbundle By Name(w734) -> ("平行样数据时间"=w733:timestamp, "平行样实测值"=w732:sgl, "平行样数据标识"=w731:string)
              }
            }
            n198 = Unbundle By Name(w664) -> ("COD跨度值"=w663:dbl)
            n199 = And(x=w671, y=u16 255) -> (x .and. y?=w672:u16)
            n200 = case shown="0, 默认" w672 {
              tunnel: ["低量程" ("格式字符串") "高量程" ("格式字符串")] -> w670
              frame 0, Default {
              }
              frame 1 {
              }
            }
            n201 = global read "VAR总磷总氮全局变量.vi" "序列号"() -> (w669:string)
            n202 = Bundle By Name(cluster=w666, "时间标识"=w677, "监测值"=w676, "数据标识"=w675, "测量模式"=w667, "单位"=w691, "因子编码"=w690, "标样参考值"=w674, "F0"=w689, "F1"=w688, "F2"=w687, "F3"=w686, "F4"=w685, "F5"=w684, "F6"=w683, "F7"=w682, "X"=w681, "温度"=w680, "湿度"=w679, "量程标识"=w670, "SN"=w669, "数据标记表"=w668, "跨度值"=w663) -> (w665:T3)
            n203 = global read "VAR总磷总氮全局变量.vi" "CODcr关键参数"() -> (w658:T9)
            n204 = call "总磷氨氮插入数据.vi"("table"=w661, "关键参数"=w658, "data"=w665) -> ()  [unwired: 12 in, 1 out]
          }
        }
      }
    }
  }
